vi "Tag.read_lua.vi"(5 "LuaVIEW reference":T1) -> (15 "error out":errorcluster)   [LabVIEW 2012]
doc: "Attempts to read the point located at the tag object's read_index from the tag's in-memory buffer. When available, the read_index attribute is incremented to the next point. Typical use is for reading points written to a tag without skipping a point. To do so, set up a loop that calls this method. The loop should stop and sleep for a bit when no more points are available.\nParameters:\nobj:tag\nResults:\nnum:value, value of the read point. NaN if not available.\nnum:time, timestamp of the read point. NaN if not available.\nbool:available, false when the point is not yet available.\nErrors:\nIndexed point is no longer present in the circular tag buffer.\nInvalid or dead tag object.\nData logger not initialized."
uses:
  luaview/typedefs/t_LuaVIEW Reference.ctl
  typedefs/t_DataLog Tag Buffers Methods.ctl
  luaview/subvis/private/LuaVIEW Pull (object).vi
  luaview/subvis/private/LuaVIEW Pull (I32).vi
  luaview/subvis/private/LuaVIEW Push (number).vi
  luaview/subvis/private/LuaVIEW Push (boolean).vi
  luaview/subvis/private/LuaVIEW Push (I32).vi
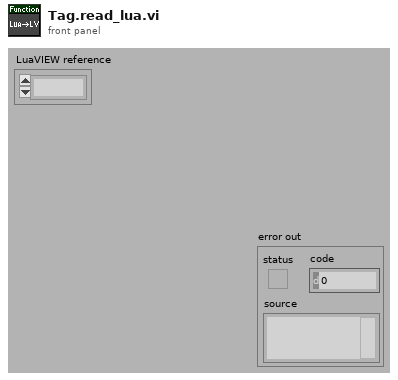
[diagram p1: front panel]
types:
  T1 = typedef "t_LuaVIEW Reference.ctl" = refnum<k1>
  T2 = typedef "t_DataLog Tag Buffers Methods.ctl" = enum16{"initialize", "inert", "write", "read", "read oldest", "read last", "cleanup"}
  T3 = typedef "t_DataLog Point.ctl" = cluster{"time":dbl, "value":dbl}
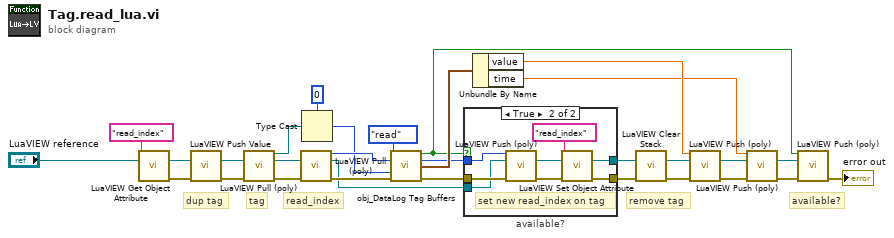
[diagram p0: block diagram]
diagram:
  # "dup tag"
  # "remove tag"
  # "available?"
  # "tag"
  # "read_index"
  n1 = call "LuaVIEW Get Object Attribute.vi"("key"="read_index", "LuaVIEW reference in"="LuaVIEW reference") -> ("LuaVIEW reference out"=w10:T1, "error out"=w11:errorcluster)  [unwired: 12 in]
  n2 = call "LuaVIEW Push Value.vi"("LuaVIEW reference in"=w10, "error in (no error)"=w11) -> ("LuaVIEW reference out"=w9:T1, "error out"=w8:errorcluster)  [unwired: 12 in]
  n3 = call-poly "LuaVIEW Pull (poly).vi"("LuaVIEW reference in"=w9, "error in (no error)"=w8) -> ("object refnum"=w21:refnum<vi>, "LuaVIEW reference out"=w15:T1, "error out"=w19:errorcluster)  [unwired: 10 in, 1 out]
  n4 = call-poly "LuaVIEW Pull (poly).vi"("LuaVIEW reference in"=w15, "error in (no error)"=w19) -> ("I32"=w24:i32, "LuaVIEW reference out"=w13:T1, "error out"=w23:errorcluster)  [unwired: 11 in]
  n5 = Type Cast(type=0 ("read index in"), x=w21) -> (*(type *) &x=w18:i32)
  n6 = call "obj_DataLog Tag Buffers.vi"("method"=t_DataLog_Tag_Buffers_Methods."read", "read index in"=w24, "tag index"=w18, "error in (no error)"=w23) -> ("available?"=w5:bool, "read index out"=w12:i32, "point out"=w29:T3, "error out"=w14:errorcluster)  [unwired: 7 in, 1 out]
  n7 = case "available?" shown="True" w5 {
    tunnel: w14 -> [w31 w40]
    tunnel: w13 -> [w32 w38]
    tunnel: w12 -> [_ w36]
    tunnel: [w31 w34] -> w4
    tunnel: [w32 w33] -> w3
    frame False {
    }
    frame True {
      # "set new read_index on tag"
      n8 = call-poly "LuaVIEW Push (poly).vi"("I32"=w36, "LuaVIEW reference in"=w38, "error in (no error)"=w40) -> ("LuaVIEW reference out"=w37:T1, "error out"=w39:errorcluster)  [unwired: 11 in]
      n9 = call "LuaVIEW Set Object Attribute.vi"("key"="read_index", "LuaVIEW reference in"=w37, "error in (no error)"=w39) -> ("LuaVIEW reference out"=w33:T1, "error out"=w34:errorcluster)  [unwired: 11 in]
    }
  }
  n10 = Unbundle By Name(w29) -> ("value"=w27:dbl, "time"=w26:dbl)
  n11 = call "LuaVIEW Clear Stack.vi"("LuaVIEW reference in"=w3, "error in (no error)"=w4) -> ("LuaVIEW reference out"=w2:T1, "error out"=w1:errorcluster)  [unwired: 12 in]
  n12 = call-poly "LuaVIEW Push (poly).vi"("number"=w27, "LuaVIEW reference in"=w2, "error in (no error)"=w1) -> ("LuaVIEW reference out"=w28:T1, "error out"=w25:errorcluster)  [unwired: 11 in]
  n13 = call-poly "LuaVIEW Push (poly).vi"("number"=w26, "LuaVIEW reference in"=w28, "error in (no error)"=w25) -> ("LuaVIEW reference out"=w6:T1, "error out"=w7:errorcluster)  [unwired: 11 in]
  n14 = call-poly "LuaVIEW Push (poly).vi"("boolean"=w5, "LuaVIEW reference in"=w6, "error in (no error)"=w7) -> ("error out"=→"error out":errorcluster)  [unwired: 11 in, 1 out]
